vi "setup Write Servo LV.vi"(9 "value":u16, 10 "servoNum":u8, 11 "instance":i32) -> ()   [LabVIEW 2022 SP3, in "SADI_FW3.lvlib"]
doc: "SADI_API_Wrapper void setupWrite_Servo_LV( int instance ,\n uint8_t servoNum ,\n uint16_t value );"
uses:
  SADI_FW3.lvlib
  SADI_FW3.dll
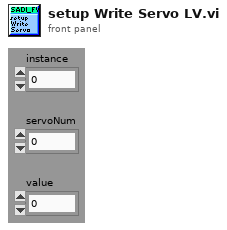
[diagram p1: front panel]
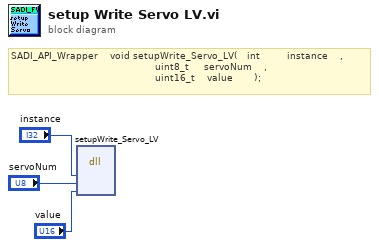
[diagram p0: block diagram]
diagram:
  # "SADI_API_Wrapper    void setupWrite_Servo_LV(   int         instance    ,\n                                                uint8_t     servoNum    ,\n                                                uint16_t    value       );"
  n1 = dll-call lib="C:/Users/scer/OneDrive - University of Florida/eml4314c/eml4314SP23/resources/release_2_3_23/LV/LVLib/SADI_FW3.*" fn="setupWrite_Servo_LV"("instance"="instance", "servoNum"="servoNum", "value"="value") -> ()  [unwired: 7 in, 2 out]
